vi "Num Ref Check Value Valid.vi"(8 "error in":errorcluster, 11 "Num Ref":refnum<vi>) -> (0 "error out":errorcluster, 3 "Valid":bool)   [LabVIEW 2018, in "Main Panel.lvlib" / "Main Panel.lvclass"]
uses:
  Main Panel.lvclass
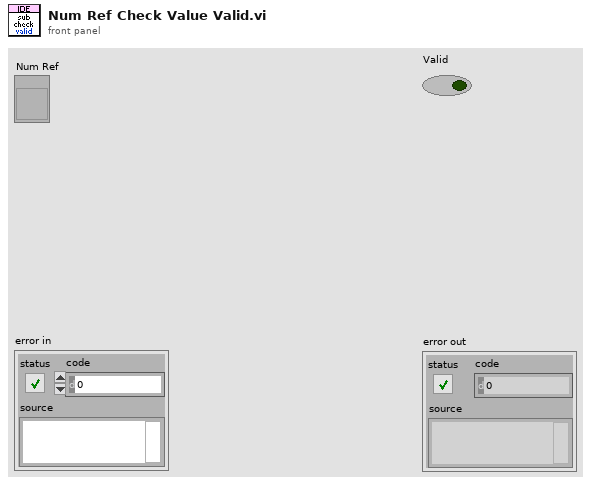
[diagram p1: front panel]
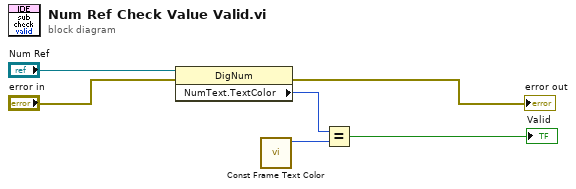
[diagram p0: block diagram]
diagram:
  n1 = property class="DigNum"(reference="Num Ref", error in="error in") -> (error out=→"error out":errorcluster, "NumText.TextColor"=w3:u32)  [unwired: 1 out]
  n2 = call "Const Frame Text Color.vi"() -> ("valid num color"=w2:u32)  [unwired: 10 in, 1 out]
  n3 = Equal?(x=w3, y=w2) -> (x = y?=→"Valid":bool)
